vi "Plotting Location.vi"(5 "Z Adaption":dbl, 6 "Refresh Rate (ms)":dbl, 7 "Angle":dbl, 8 "Y-Motion":dbl, 9 "Old Y":dbl, 10 "Old X":dbl, 11 "X-Motion":dbl) -> (1 "New Y":dbl, 2 "New X":dbl)   [LabVIEW 2015]
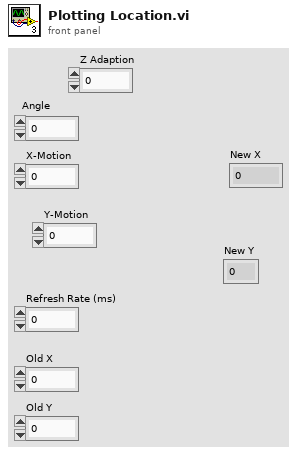
[diagram p1: front panel]
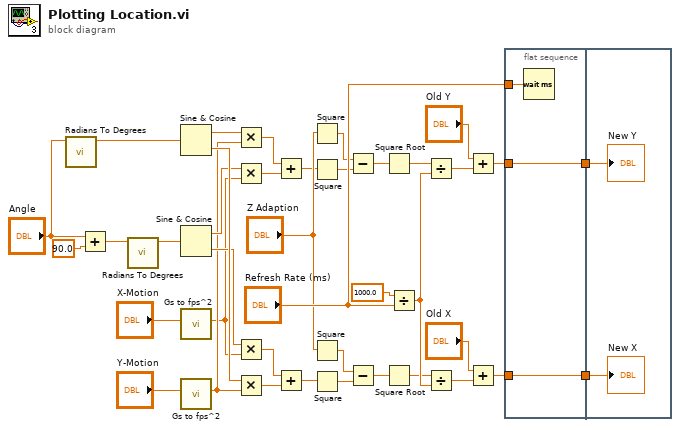
[diagram p0: block diagram]
diagram:
  n1 = call "Radians To Degrees.vi"("Degrees"="Angle") -> ("Radians"=w35:dbl)  [unwired: 10 in]
  n2 = Add(x="Angle", y=90.0) -> (x+y=w33:dbl)
  n3 = call "Radians To Degrees.vi"("Degrees"=w33) -> ("Radians"=w34:dbl)  [unwired: 10 in]
  n4 = Sine & Cosine(0:w35) -> (1:w30:dbl, 2:w29:dbl)
  n5 = Sine & Cosine(0:w34) -> (1:w28:dbl, 2:w27:dbl)
  n6 = call "Gs to fps^2.vi"("g"="X-Motion") -> ("f/s^2"=w12:dbl)  [unwired: 10 in]
  n7 = call "Gs to fps^2.vi"("g"="Y-Motion") -> ("f/s^2"=w14:dbl)  [unwired: 10 in]
  n8 = Multiply(x=w30, y=w14) -> (x*y=w24:dbl)
  n9 = Multiply(x=w28, y=w12) -> (x*y=w23:dbl)
  n10 = Multiply(x=w27, y=w12) -> (x*y=w22:dbl)
  n11 = Multiply(x=w29, y=w14) -> (x*y=w21:dbl)
  n12 = Add(x=w24, y=w23) -> (x+y=w4:dbl)
  n13 = Add(x=w22, y=w21) -> (x+y=w1:dbl)
  n14 = Square(x="Z Adaption") -> (x^2=w8:dbl)
  n15 = Square(x=w4) -> (x^2=w7:dbl)
  n16 = Square(x="Z Adaption") -> (x^2=w11:dbl)
  n17 = Square(x=w1) -> (x^2=w10:dbl)
  n18 = Subtract(x=w8, y=w7) -> (x-y=w6:dbl)
  n19 = Subtract(x=w11, y=w10) -> (x-y=w9:dbl)
  n20 = Square Root(x=w6) -> (sqrt(x)=w3:dbl)
  n21 = Square Root(x=w9) -> (sqrt(x)=w2:dbl)
  n22 = Divide(x=1000.0, y="Refresh Rate (ms)") -> (x/y=w25:dbl)
  n23 = Divide(x=w3, y=w25) -> (x/y=w20:dbl)
  n24 = Divide(x=w2, y=w25) -> (x/y=w19:dbl)
  n25 = Add(x="Old Y", y=w20) -> (x+y=w37:dbl)
  n26 = Add(x="Old X", y=w19) -> (x+y=w36:dbl)
  n27 = flat-sequence {
    tunnel: w36 -> [w41]
    tunnel: w37 -> [w42]
    tunnel: [w42] -> w18
    tunnel: [w41] -> w17
    tunnel: "Refresh Rate (ms)" -> [w40]
    tunnel: w18 -> [w44]
    tunnel: w17 -> [w43]
    frame #0 {
      n28 = Wait (ms)(milliseconds to wait=w40) -> ()  [unwired: 1 out]
    }
    frame #1 {
      "New X" <- w43
      "New Y" <- w44
    }
  }
